vi "ConvertDLPVAGainStages_to_dB.vi"(1 "Gain_2 i":bool, 2 "Gain_1 i":bool) -> (0 "Gain (dB)":dbl)   [LabVIEW 2010]
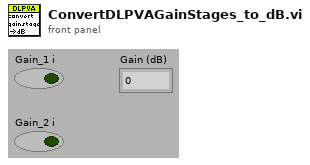
[diagram p1: front panel]
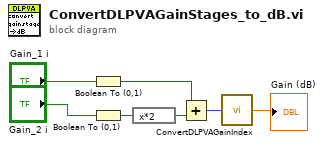
[diagram p0: block diagram]
diagram:
  n1 = Boolean To (0,1)(Boolean="Gain_1 i") -> (0, 1=w1:i16)
  n2 = Boolean To (0,1)(Boolean="Gain_2 i") -> (0, 1=w3:i16)
  n3 = expression code="x*2"(w3) -> (w2:i16)
  n4 = Add(x=w1, y=w2) -> (x+y=w4:i16)
  n5 = call "ConvertDLPVAGainIndex.vi"("Numeric 2"=w4) -> ("Numeric"=→"Gain (dB)":dbl)
